vi "At field and stable.vi"(1 "last 20 field numbers":dbl[unit][](array[numeric]), 2 "Desired field":dbl[unit]) -> (0 "At field and stable?":bool)   [LabVIEW 2009, in "Varian.lvlib"]
uses:
  Varian.lvlib
  <vilib>/Analysis/NI_AALBase.lvlib
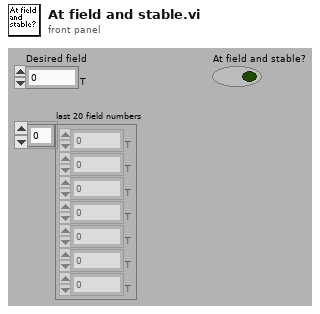
[diagram p1: front panel]
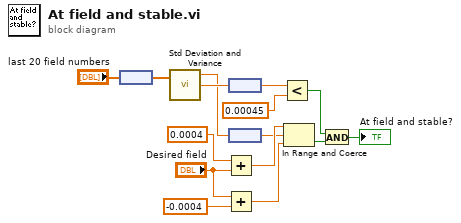
[diagram p0: block diagram]
diagram:
  n1 = node("last 20 field numbers") -> (w3:dbl[])
  n2 = call <vilib>:"Std Deviation and Variance.vi"("X"=w3) -> ("mean"=w10:dbl, "standard deviation"=w12:dbl)  [unwired: 1 in, 1 out]
  n3 = Add(x=dbl[unit] 0.0004, y="Desired field") -> (x+y=w5:dbl[unit])
  n4 = Add(x="Desired field", y=dbl[unit] -0.0004) -> (x+y=w6:dbl[unit])
  n5 = node(w12) -> (w1:dbl[unit])
  n6 = node(w10) -> (w2:dbl[unit])
  n7 = Less?(x=w1, y=dbl[unit] 0.00045 ("x")) -> (x < y?=w13:bool)
  n8 = In Range and Coerce(upper limit=w5, x=w2, lower limit=w6) -> (In Range?=w14:bool)  [unwired: 1 out]
  n9 = And(x=w13, y=w14) -> (x .and. y?=→"At field and stable?":bool)
